vi "Constant wfmTermValue.vi"() -> (0 "wfm end value":u64)   [LabVIEW 2018]
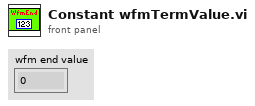
[diagram p1: front panel]
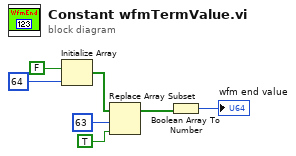
[diagram p0: block diagram]
diagram:
  n1 = Initialize Array(FALSE, 64 ("dimension size")) -> (w5:bool[])
  n2 = Replace Array Subset(array=w5, new element=TRUE, index=63) -> (w2:bool[])
  n3 = Boolean Array To Number(Boolean array=w2) -> (number=→"wfm end value":u64)
